vi "My_IP.vi"() -> ()   [LabVIEW 2010]
panel:
  in  "dot notation? (F)":bool
  out "name":string
  out "net address":u32
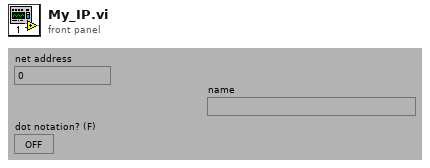
[diagram p1: front panel]
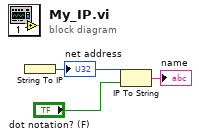
[diagram p0: block diagram]
diagram:
  n1 = String To IP() -> (0:w3:u32)  [unwired: 1 out]
  "net address" <- w3
  n2 = IP To String(1:"dot notation? (F)", 2:w3) -> (0:→"name":string)
